vi "Run.vi"(8 "error in (no error)":errorcluster, 11 "LUnit Test Suite In":refnum<class "LUnit Test Suite.lvclass">) -> (0 "error out":errorcluster, 1 "Done?":bool, 2 "Results":T1[](array[typedef]), 3 "LUnit Test Suite Out":refnum<class "LUnit Test Suite.lvclass">)   [LabVIEW 2020, in "LUnit Test Suite.lvclass"]
doc: "Execute next test in suite. Done indicator is True if the test suite is exhausted and all active tests have been run."
uses:
  LUnit Test Suite.lvclass
  Result/Result.ctl
  Result/Status.ctl
  Result/Type.ctl
  LUnit Test Suite.lvclass/LUnit Test Suite.ctl
  Runnable.lvclass
  Result/Result.lvlib
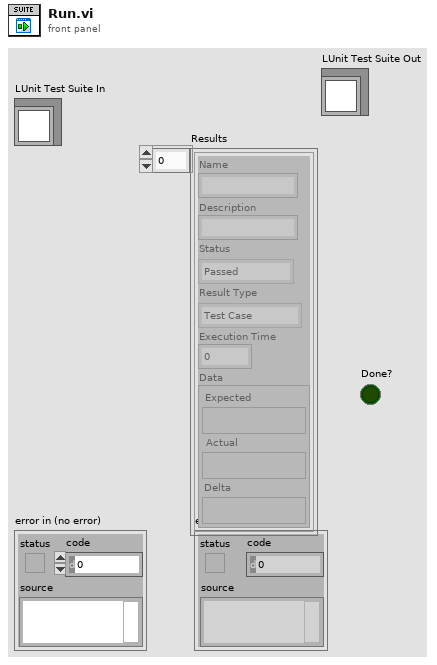
[diagram p1: front panel]
types:
  T1 = typedef "Result.lvlib/Result.ctl" = cluster{"Name":string, "Description":string, "Status":T2, "Result Type":T3, "Execution Time":dbl, "Data":cluster{"Expected":variant, "Actual":variant, "Delta":variant}}
  T2 = typedef "Result.lvlib/Status.ctl" = enum16{"", "Passed", "Failed", "Error", "Skipped", "Setup Error", "Broken", "Teardown Error"}
  T3 = typedef "Result.lvlib/Type.ctl" = enum16{"Test Case", "Test Suite", "Test Run", "Pass", "Fail", "Skip", "Pass if", "Fail if", "Pass if Error", "Fail if Error", "Pass if Equal", "Fail if Equal"}
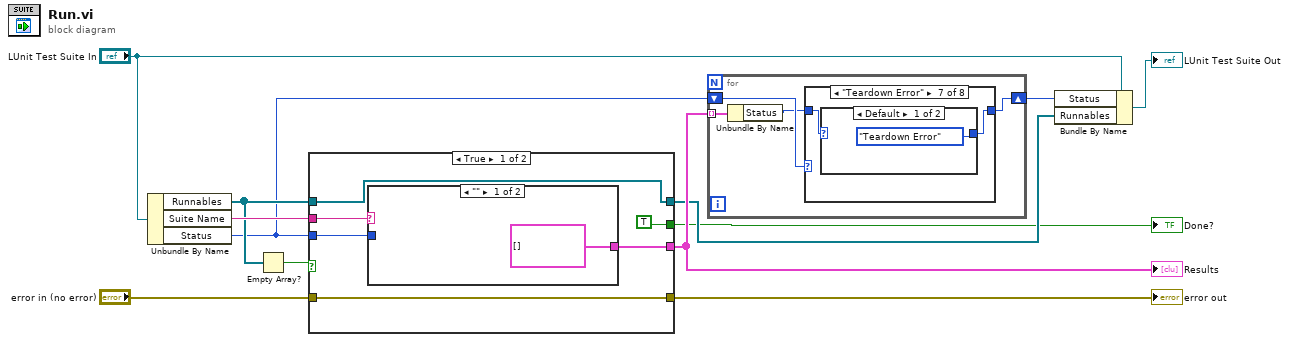
[diagram p0: block diagram]
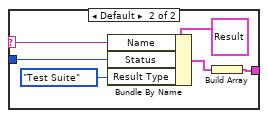
[diagram p2: hidden frame]
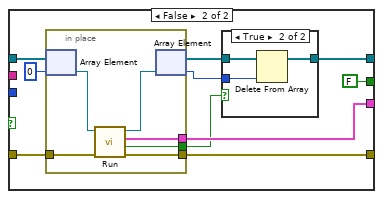
[diagram p3: hidden frame]
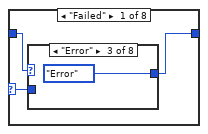
[diagram p5: hidden frame]
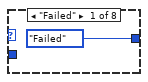
[diagram p6: hidden frame]
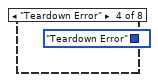
[diagram p8: hidden frame]
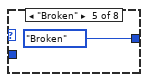
[diagram p9: hidden frame]
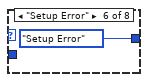
[diagram p10: hidden frame]
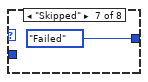
[diagram p11: hidden frame]
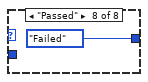
[diagram p12: hidden frame]
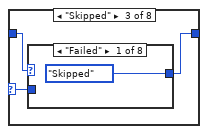
[diagram p14: hidden frame]
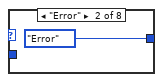
[diagram p15: hidden frame]
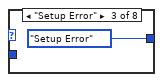
[diagram p16: hidden frame]
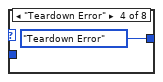
[diagram p17: hidden frame]
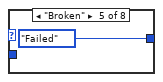
[diagram p18: hidden frame]
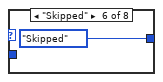
[diagram p19: hidden frame]
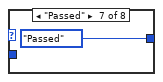
[diagram p20: hidden frame]
diagram:
  n1 = Unbundle By Name("LUnit Test Suite In") -> ("Runnables"=w3:refnum<class "Runnable.lvclass">[], "Suite Name"=w4:string, "Status"=w2:T2)
  n2 = Empty Array?(array=w3) -> (empty?=w1:bool)
  n3 = case shown="True" w1 {
    tunnel: "error in (no error)" -> [w16 w35]
    tunnel: [w16 w34] -> w11
    tunnel: w3 -> [w18 w31]
    tunnel: [w17 w33] -> w8
    tunnel: [w18 w27] -> w7
    tunnel: [TRUE FALSE] -> w6
    tunnel: w4 -> [w14 _]
    tunnel: w2 -> [w13 _]
    frame True {
      n4 = case shown="\"\"" w14 {
        selector: w14 -> [_ w24]
        tunnel: w13 -> [_ w23]
        tunnel: [T1[] [] w21] -> w17
        frame "" {
        }
        frame Default {
          n5 = Bundle By Name(cluster=T1 {"Name"="", "Description"="", "Status"=enum."Passed", "Result Type"=enum."Test Case", "Execution Time"=0.0, "Data"={"Expected"=variant, "Actual"=variant, "Delta"=variant}} ("Results"), "Name"=w24, "Status"=w23, "Result Type"=Type."Test Suite") -> (w22:T1)
          n6 = Build Array(w22) -> (w21:T1[])
        }
      }
    }
    frame False {
      n7 = in-place {
        in-place-border: w35 -> [w45]
        in-place-border: [w44] -> w34
        in-place-border: [w43] -> w33
        in-place-border: [w40] -> w26
        n8 = in-place-array #1(w31, 0) -> (w42:refnum<class "Runnable.lvclass">)
        n9 = call-dynamic "Run.vi"("error in (no error)"=w45, "Runnable In"=w42) -> ("error out"=w44:errorcluster, "Done?"=w40:bool, "Results"=w43:T1[], "Runnable Out"=w41:refnum<class "Runnable.lvclass">)  [unwired: 6 in]
        n10 = in-place-array #1(w41) -> (w28:refnum<class "Runnable.lvclass">[], w29:i32)
      }
      n11 = case shown="True" w26 {
        tunnel: w29 -> [_ w39]
        tunnel: w28 -> [w36 w38]
        tunnel: [w36 w37] -> w27
        frame False {
        }
        frame True {
          n12 = Delete From Array(array=w38, index=w39) -> (array with subset deleted=w37:refnum<class "Runnable.lvclass">[])  [unwired: 1 in, 1 out]
        }
      }
    }
  }
  "error out" <- w11
  "Results" <- w8
  "Done?" <- w6
  n13 = for {
    shift-right: [w48] -> w9
    shift-left: w2 -> [w49]
    tunnel: w8 -> [w47] mode=indexing
    n14 = Unbundle By Name(w47) -> ("Status"=w46:T2)
    n15 = case shown="\"Teardown Error\"" w49 {
      selector: w49 -> [w50 _ w62 w73 _ _ _ _]
      tunnel: w46 -> [w52 w61 w64 w75 _ _ w86 w90]
      tunnel: [w51 w61 w63 w74 Status."Error" ("Merged Status") Status."Setup Error" ("Merged Status") w87 w90] -> w48
      frame "Failed" {
        n16 = case shown="\"Error\"" w52 {
          tunnel: [Status."Failed" ("Merged Status") w54 Status."Error" ("Merged Status") Status."Teardown Error" ("Merged Status") Status."Broken" ("Merged Status") Status."Setup Error" ("Merged Status") Status."Failed" ("Merged Status") Status."Failed" ("Merged Status")] -> w51
          tunnel: w50 -> [_ w54 _ _ _ _ _ _]
          frame "Failed" {
          }
          frame "" {
          }
          frame "Error" {
          }
          frame "Teardown Error" {
          }
          frame "Broken" {
          }
          frame "Setup Error" {
          }
          frame "Skipped" {
          }
          frame "Passed" {
          }
        }
      }
      frame "" {
      }
      frame "Skipped" {
        n17 = case shown="\"Failed\"" w64 {
          tunnel: [Status."Skipped" ("Merged Status") Status."Error" ("Merged Status") Status."Setup Error" ("Merged Status") Status."Teardown Error" ("Merged Status") Status."Failed" ("Merged Status") Status."Skipped" ("Merged Status") Status."Passed" ("Merged Status") w72] -> w63
          tunnel: w62 -> [_ _ _ _ _ _ _ w72]
          frame "Failed" {
          }
          frame "Error" {
          }
          frame "Setup Error" {
          }
          frame "Teardown Error" {
          }
          frame "Broken" {
          }
          frame "Skipped" {
          }
          frame "Passed" {
          }
          frame "" {
          }
        }
      }
      frame "Passed" {
        n18 = case shown="\"Teardown Error\"" w75 {
          tunnel: [Status."Failed" ("Merged Status") Status."Error" ("Merged Status") Status."Setup Error" ("Merged Status") Status."Failed" ("Merged Status") Status."Teardown Error" ("Merged Status") Status."Passed" ("Merged Status") w82 Status."Passed" ("Merged Status")] -> w74
          tunnel: w73 -> [_ _ _ _ _ _ w82 _]
          frame "Failed" {
          }
          frame "Error" {
          }
          frame "Setup Error" {
          }
          frame "Broken" {
          }
          frame "Teardown Error" {
          }
          frame "Skipped" {
          }
          frame "" {
          }
          frame "Passed" {
          }
        }
      }
      frame "Error" {
      }
      frame "Setup Error" {
      }
      frame "Teardown Error" {
        n19 = case shown="Default" w86 {
          selector: w86 -> [_ w89]
          tunnel: [Status."Teardown Error" ("Merged Status") w89] -> w87
          frame Default {
          }
          frame "Error", "Setup Error", "Broken" {
          }
        }
      }
      frame "Broken" {
      }
    }
  }
  n20 = Bundle By Name(cluster="LUnit Test Suite In", "Status"=w9, "Runnables"=w7) -> (→"LUnit Test Suite Out":refnum<class "LUnit Test Suite.lvclass">)
